vi "Import Scalars - all.vi"(8 "error in":errorcluster, 11 "FPGA addon refnum in":T3=18446744073709551615 format="%.0x") -> (0 "error out":errorcluster, 2 "imported bitfile scalars out":T1[](array[typedef]), 3 "FPGA addon refnum out":T3=18446744073709551615 format="%.0x")   [LabVIEW 2018, in "Scripting API.lvlib"]
uses:
  Scripting API.lvlib
  <vilib>/NI Veristand/Custom Device API/Custom Device Item Ref.ctl
  TypeDefs/Output Scalar Data.ctl
  Addon/Addon Shared/Types/Data Type.ctl
  Addon/Addon System Explorer/Types/Channel Type.ctl
  Addon/Addon Shared/Types/FG Action.ctl
  Addon/Addon Shared/SubVIs/Constants.vi
  <vilib>/NI/NI VeriStand Advanced SysDef API/_SubVIs/SysDef.Search.GUID.vi
  <vilib>/NI/NI VeriStand Advanced SysDef API/SysDef API/SysDef.Property.Get.vi
  <vilib>/NI/NI VeriStand Advanced SysDef API/_SubVIs/SysDef.Property.Get.Variant.vi
  <vilib>/NI/NI VeriStand Advanced SysDef API/SysDef API/SysDef.Property.Set.vi
  <vilib>/NI/NI VeriStand Advanced SysDef API/_SubVIs/SysDef.Property.Set.Variant.vi
  Addon/Addon Shared/FPGA Addon Shared.lvlib
  <vilib>/NI/NI VeriStand Advanced SysDef API/SysDef API/Advanced System Definition.lvlib
  Addon/Addon System Explorer/FPGA Addon System Explorer.lvlib
  <vilib>/NI Veristand/Custom Device API/Custom Device API.lvlib
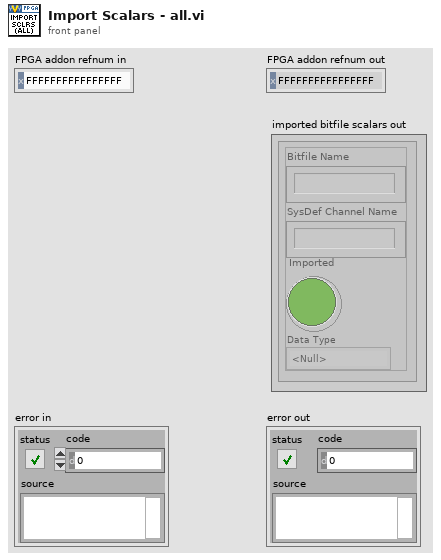
[diagram p1: front panel]
types:
  T1 = typedef "Scripting API.lvlib/Output Scalar Data.ctl" = cluster{"Bitfile Name":string, "SysDef Channel Name":string, "Imported":bool, "Data Type":T2}
  T2 = typedef "FPGA Addon Shared.lvlib/Data Type.ctl" = enum8{"<Null>", "I8", "I16", "I32", "I64", "U8", "U16", "U32", "U64", "SGL", "Boolean", "Analog PWM In Settings", "Analog PWM In", "Digital PWM In Settings", "Digital PWM In", "Digital PWM Out", "Sine Out", "FXP+/-24.5", "FXP+/-16.5", "FXP+/-32.8", "FXP+/-64.32", "FXP+/-16.7", "FXP+/-20.5", "FXP+/-27.5", "FXP+/-32.16", "FXP+16.3", "FXP+18.3", "Digital Static In", "Digital Static Out", "Digital Static In Settings", "Digital WSS Out", "Quad Encoder Settings", "Quad Encoder In", "Group"}
  T3 = typedef "Custom Device API.lvlib/Custom Device Item Ref.ctl" = u64
  T4 = typedef "FPGA Addon System Explorer.lvlib/Channel Type.ctl" = enum16{"Write Channel", "Read Channel", "Write Waveform", "Read Waveform"}
  T5 = typedef "FPGA Addon Shared.lvlib/FG Action.ctl" = enum8{"GET", "SET"}
  T6 = typedef "FPGA Addon Shared.lvlib/Register Information.ctl" = cluster{"Name":string, "Data Type":T2, "Default Value":variant}
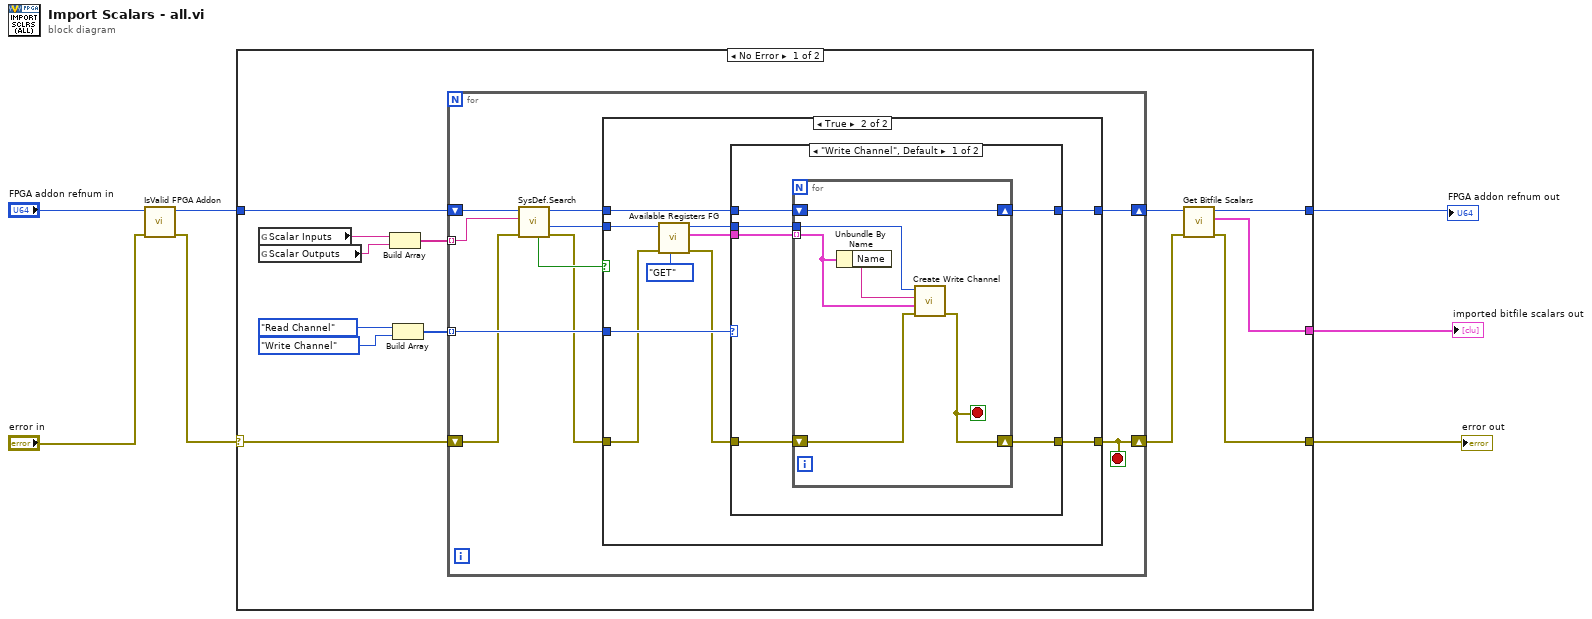
[diagram p0: block diagram]
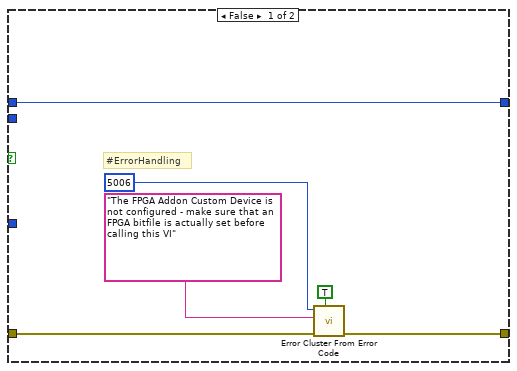
[diagram p2: hidden frame]
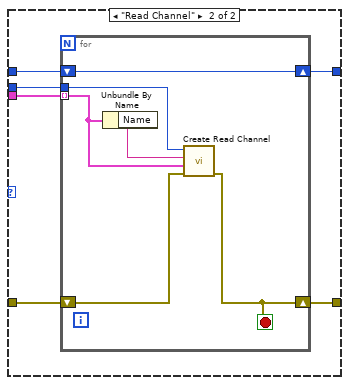
[diagram p3: hidden frame]
diagram:
  n1 = call "IsValid FPGA Addon.vi"("error in"="error in", "FPGA Addon refnum in"="FPGA addon refnum in") -> ("error out"=w5:errorcluster, "FPGA Addon refnum out"=w4:T3)  [unwired: 8 in]
  n2 = case shown="No Error" w5 {
    selector: w5 -> [w13 w72]
    tunnel: w4 -> [w18 w71]
    tunnel: [w11 w71] -> w3
    tunnel: [w9 w72] -> w2
    tunnel: [w8 _] -> w1
    frame No Error {
      n3 = global read "Constants.vi" "Scalar Inputs"() -> (w20:string)
      n4 = global read "Constants.vi" "Scalar Outputs"() -> (w19:string)
      n5 = Build Array(w20, w19) -> (w17:string[])
      n6 = Build Array(Channel_Type."Read Channel" ("Action"), Channel_Type."Write Channel" ("Action")) -> (w14:T4[])
      n7 = for {
        tunnel: w17 -> [w29] mode=indexing
        shift-right: [w22] -> w12
        shift-left: w18 -> [w30]
        tunnel: w14 -> [w26] mode=indexing
        shift-right: [w21] -> w10
        shift-left: w13 -> [w25]
        stop <- w21 stop-if-true
        n8 = call-poly <vilib>:"SysDef.Search.vi"("error in (no error)"=w25, "GUID"=w29, "nodeID"=w30) -> ("error out"=w24:errorcluster, "Value out"=w27:u64, "nodeID out"=w23:u64, "Found?"=w28:bool)  [unwired: 5 in]
        n9 = case shown="True" w28 {
          tunnel: w27 -> [_ w45]
          tunnel: w26 -> [_ w42]
          tunnel: w24 -> [w33 w41]
          tunnel: [w32 w39] -> w21
          tunnel: w23 -> [w36 w38]
          tunnel: [w36 w37] -> w22
          frame False {
            # "#ErrorHandling"
            n10 = call <vilib>:"Error Cluster From Error Code.vi"("show call chain? (False)"=TRUE, "error in (no error)"=w33, "error message (\"\")"="The FPGA Addon Custom Device is not configured - make sure that an FPGA bitfile is actually set before calling this VI" ("error message (\"\")"), "error code (0)"=5006) -> ("error out"=w32:errorcluster)  [unwired: 5 in]
          }
          frame True {
            n11 = call "Available Registers FG.vi"("Action"=FG_Action."GET", "error in (no error)"=w41, "Item Ref"=w45) -> ("error out"=w40:errorcluster, "Available Registers"=w44:T6[], "Item Ref out"=w43:T3)  [unwired: 6 in]
            n12 = case shown="\"Write Channel\", Default" w42 {
              tunnel: w44 -> [w49 w64]
              tunnel: w43 -> [w50 w63]
              tunnel: w40 -> [w52 w62]
              tunnel: [w51 w61] -> w39
              tunnel: w38 -> [w48 w60]
              tunnel: [w47 w59] -> w37
              frame "Write Channel", Default {
                n13 = for {
                  tunnel: w49 -> [w56] mode=indexing
                  tunnel: w50 -> [w58]
                  shift-right: [w53] -> w51
                  shift-left: w52 -> [w55]
                  shift-right: [w54] -> w47
                  shift-left: w48 -> [w54]
                  stop <- w53 stop-if-true
                  n14 = Unbundle By Name(w56) -> ("Name"=w57:string)
                  n15 = call "Create Write Channel.vi"("error in (no error)"=w55, "Cluster"=w56, "Bitfile Name"=w57, "Item Ref in"=w58) -> ("error out"=w53:errorcluster)  [unwired: 7 in]
                }
              }
              frame "Read Channel" {
                n16 = for {
                  tunnel: w64 -> [w68] mode=indexing
                  tunnel: w63 -> [w69]
                  shift-right: [w65] -> w61
                  shift-left: w62 -> [w67]
                  shift-right: [w66] -> w59
                  shift-left: w60 -> [w66]
                  stop <- w65 stop-if-true
                  n17 = Unbundle By Name(w68) -> ("Name"=w70:string)
                  n18 = call "Create Read Channel.vi"("error in (no error)"=w67, "Channel"=w68, "Bitfile Name"=w70, "Item Ref in"=w69) -> ("error out"=w65:errorcluster)  [unwired: 7 in]
                }
              }
            }
          }
        }
      }
      n19 = call "Get Bitfile Scalars.vi"("error in"=w10, "FPGA addon refnum in"=w12) -> ("error out"=w9:errorcluster, "bitfile scalars out"=w8:T1[], "FPGA addon refnum out"=w11:T3)  [unwired: 7 in]
    }
    frame Error {
    }
  }
  "error out" <- w2
  "FPGA addon refnum out" <- w3
  "imported bitfile scalars out" <- w1
